vi "MeasureDarkCurrent.vi"(8 "Multimeter GPIB Address":string, 9 "Amplifier":refnum<visa-resource-name>) -> (0 "Amplifier Error":errorcluster, 1 "Amplifier Settings":T1)   [LabVIEW 2017]
uses:
  Linear Dichroism Controller/AmplifierSettings.ctl
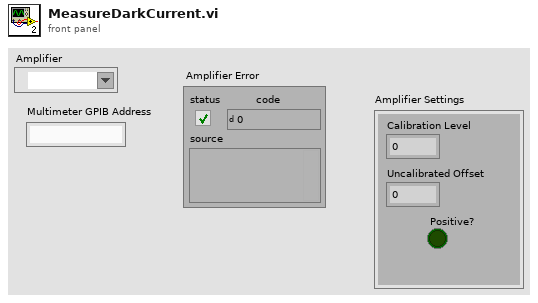
[diagram p1: front panel]
types:
  T1 = typedef "AmplifierSettings.ctl" = cluster{"Calibration Level":dbl, "Uncalibrated Offset":dbl, "Positive?":bool}
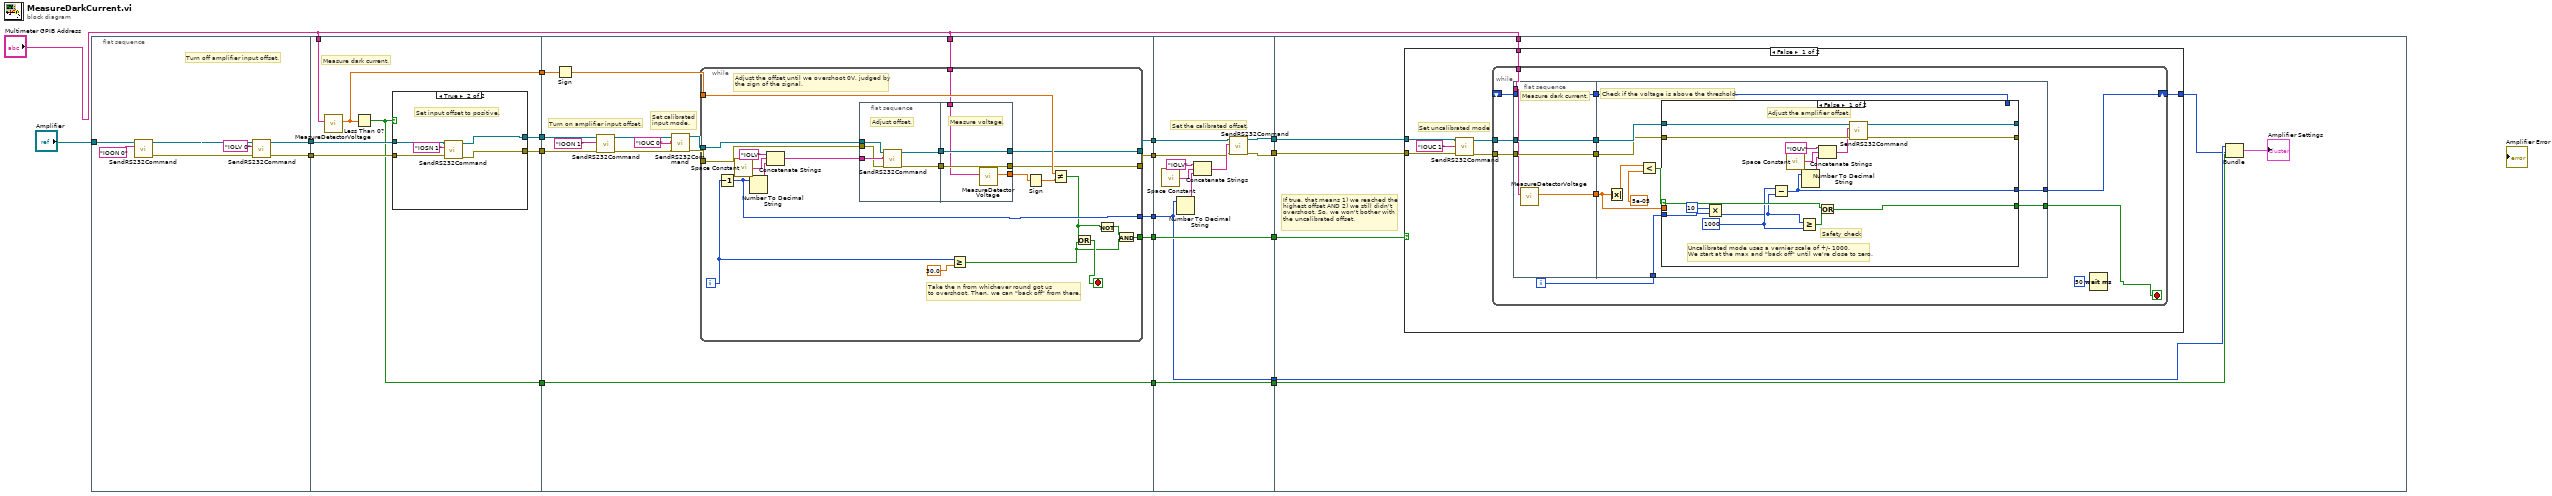
[diagram p0: block diagram]
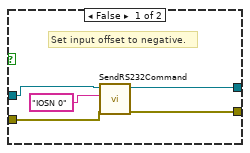
[diagram p2: hidden frame]
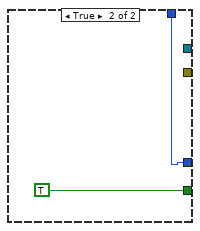
[diagram p3: hidden frame]
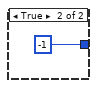
[diagram p4: hidden frame]
diagram:
  n1 = flat-sequence {
    tunnel: "Amplifier" -> [w25]
    tunnel: [w23] -> w17
    tunnel: [w22] -> w16
    tunnel: w17 -> [w32]
    tunnel: w16 -> [w31]
    tunnel: [w30] -> w15
    tunnel: [w29] -> w14
    tunnel: [w28] -> w13
    tunnel: "Multimeter GPIB Address" -> [w27]
    tunnel: [w26] -> w1
    tunnel: w15 -> [w57]
    tunnel: w14 -> [w56]
    tunnel: w13 -> [w55]
    tunnel: [w53] -> w12
    tunnel: [w52] -> w11
    tunnel: [w51] -> w10
    tunnel: [w45] -> w6
    tunnel: "Multimeter GPIB Address" -> [w44]
    tunnel: [w43] -> w2
    tunnel: w1 -> [w43]
    tunnel: w12 -> [w95]
    tunnel: w11 -> [w96]
    tunnel: w10 -> [w91]
    tunnel: [w94] -> w9
    tunnel: [w93] -> w8
    tunnel: [w92] -> w7
    tunnel: w6 -> [w92]
    tunnel: [w91] -> w4
    tunnel: [w90] -> w3
    tunnel: w2 -> [w90]
    tunnel: w9 -> [w107]
    tunnel: w8 -> [w108]
    tunnel: w7 -> [w106]
    tunnel: "Multimeter GPIB Address" -> [w105]
    tunnel: w4 -> [w104]
    tunnel: w3 -> [w102]
    frame #0 {
      # "Turn off amplifier input offset."
      n2 = call "SendRS232Command.vi"("Command"="IOON 0", "VISA/RS232 Device In"=w25) -> ("error out"=w20:errorcluster, "VISA/RS232 Device Out"=w21:refnum<visa-resource-name>)  [unwired: 8 in]
      n3 = call "SendRS232Command.vi"("error in (no error)"=w20, "Command"="IOLV 0", "VISA/RS232 Device In"=w21) -> ("error out"=w22:errorcluster, "VISA/RS232 Device Out"=w23:refnum<visa-resource-name>)  [unwired: 7 in]
    }
    frame #1 {
      # "Measure dark current."
      n4 = call "MeasureDetectorVoltage.vi"("GPIB Address"=w27) -> ("Average Voltage"=w28:dbl)  [unwired: 10 in]
      n5 = Less Than 0?(x=w28) -> (x < 0?=w26:bool)
      n6 = case shown="True" w26 {
        tunnel: w32 -> [w36 w42]
        tunnel: w31 -> [w35 w41]
        tunnel: [w34 w39] -> w30
        tunnel: [w33 w38] -> w29
        frame False {
          # "Set input offset to negative."
          n7 = call "SendRS232Command.vi"("error in (no error)"=w35, "Command"="IOSN 0", "VISA/RS232 Device In"=w36) -> ("error out"=w33:errorcluster, "VISA/RS232 Device Out"=w34:refnum<visa-resource-name>)  [unwired: 7 in]
        }
        frame True {
          # "Set input offset to positive."
          n8 = call "SendRS232Command.vi"("error in (no error)"=w41, "Command"="IOSN 1", "VISA/RS232 Device In"=w42) -> ("error out"=w38:errorcluster, "VISA/RS232 Device Out"=w39:refnum<visa-resource-name>)  [unwired: 7 in]
        }
      }
    }
    frame #2 {
      # "Set calibrated \ninput mode."
      # "Turn on amplifier input offset."
      n9 = Sign(1:w55) -> (0:w54:dbl)
      n10 = call "SendRS232Command.vi"("error in (no error)"=w56, "Command"="IOON 1", "VISA/RS232 Device In"=w57) -> ("error out"=w48:errorcluster, "VISA/RS232 Device Out"=w49:refnum<visa-resource-name>)  [unwired: 7 in]
      n11 = call "SendRS232Command.vi"("error in (no error)"=w48, "Command"="IOUC 0", "VISA/RS232 Device In"=w49) -> ("error out"=w46:errorcluster, "VISA/RS232 Device Out"=w47:refnum<visa-resource-name>)  [unwired: 7 in]
      n12 = while {
        tunnel: w47 -> [w76]
        tunnel: w46 -> [w75]
        tunnel: w54 -> [w71]
        tunnel: [w65] -> w51
        tunnel: [w67] -> w53
        tunnel: [w66] -> w52
        tunnel: [w60] -> w45
        tunnel: w44 -> [w59]
        i -> [w73]
        stop <- w64 stop-if-true
        # "Take the n from whichever round got us \nto overshoot. Then, we can \"back off\" from there."
        # "Adjust the offset until we overshoot 0V, judged by\nthe sign of the signal."
        n13 = Decrement(x=w73) -> (x-1=w65:i32)
        n14 = call <vilib>:"Space Constant.vi"() -> ("String"=w79:string)
        n15 = Number To Decimal String(number=w65) -> (decimal integer string=w78:string)  [unwired: 1 in]
        n16 = Concatenate Strings("IOLV", w79, w78) -> (w77:string)
        n17 = flat-sequence {
          tunnel: w77 -> [w85]
          tunnel: w76 -> [w84]
          tunnel: w75 -> [w83]
          tunnel: [w82] -> w70
          tunnel: [w81] -> w69
          tunnel: [w89] -> w68
          tunnel: w70 -> [w88]
          tunnel: w69 -> [w87]
          tunnel: [w88] -> w67
          tunnel: [w87] -> w66
          tunnel: w59 -> [w86]
          frame #0 {
            # "Adjust offset."
            n18 = call "SendRS232Command.vi"("error in (no error)"=w83, "Command"=w85, "VISA/RS232 Device In"=w84) -> ("error out"=w81:errorcluster, "VISA/RS232 Device Out"=w82:refnum<visa-resource-name>)  [unwired: 7 in]
          }
          frame #1 {
            # "Measure voltage."
            n19 = call "MeasureDetectorVoltage.vi"("GPIB Address"=w86) -> ("Average Voltage"=w89:dbl)  [unwired: 10 in]
          }
        }
        n20 = Greater Or Equal?(x=w73, y=30.0) -> (x >= y?=w61:bool)
        n21 = Sign(1:w68) -> (0:w72:dbl)
        n22 = Not Equal?(x=w71, y=w72) -> (x != y?=w63:bool)
        n23 = Or(x=w63, y=w61) -> (x .or. y?=w64:bool)
        n24 = Not(x=w63) -> (.not. x?=w62:bool)
        n25 = And(x=w62, y=w61) -> (x .and. y?=w60:bool)
      }
    }
    frame #3 {
      # "Set the calibrated offset."
      n26 = call <vilib>:"Space Constant.vi"() -> ("String"=w99:string)
      n27 = Number To Decimal String(number=w91) -> (decimal integer string=w100:string)  [unwired: 1 in]
      n28 = Concatenate Strings("IOLV", w99, w100) -> (w97:string)
      n29 = call "SendRS232Command.vi"("error in (no error)"=w96, "Command"=w97, "VISA/RS232 Device In"=w95) -> ("error out"=w94:errorcluster, "VISA/RS232 Device Out"=w93:refnum<visa-resource-name>)  [unwired: 7 in]
    }
    frame #4 {
      # "If true, that means 1) we reached the \nhighest offset AND 2) we still didn't \novershoot. So, we won't bother with \nthe uncalibrated offset."
      n30 = case shown="False" w106 {
        tunnel: w108 -> [w112 _]
        tunnel: w107 -> [w111 _]
        tunnel: w105 -> [w110 _]
        tunnel: [w109 -1] -> w103
        frame False {
          # "Set uncalibrated mode"
          n31 = call "SendRS232Command.vi"("error in (no error)"=w111, "Command"="IOUC 1", "VISA/RS232 Device In"=w112) -> ("error out"=w114:errorcluster, "VISA/RS232 Device Out"=w115:refnum<visa-resource-name>)  [unwired: 7 in]
          n32 = while {
            tunnel: w115 -> [w125]
            tunnel: w114 -> [w123]
            tunnel: w110 -> [w119]
            shift-right: [w118] -> w109
            shift-left: _ -> [w116]
            i -> [w122]
            stop <- w121 stop-if-true
            n33 = flat-sequence {
              tunnel: [w132] -> w127
              tunnel: [w131] -> w126
              tunnel: w125 -> [w131]
              tunnel: [w130] -> w124
              tunnel: w123 -> [w130]
              tunnel: w119 -> [w129]
              tunnel: [w128] -> w117
              tunnel: w116 -> [w128]
              tunnel: w127 -> [w139]
              tunnel: [w138] -> w121
              tunnel: w126 -> [w137]
              tunnel: w124 -> [w136]
              tunnel: w122 -> [w135]
              tunnel: [w134] -> w118
              tunnel: w117 -> [w133]
              frame #0 {
                # "Measure dark current."
                n34 = call "MeasureDetectorVoltage.vi"("GPIB Address"=w129) -> ("Average Voltage"=w132:dbl)  [unwired: 10 in]
              }
              frame #1 {
                # "Check if the voltage is above the threshold."
                n35 = Absolute Value(x=w139) -> (abs(x)=w142:dbl)
                n36 = Less?(x=w142, y=5e-05) -> (x < y?=w140:bool)
                n37 = case shown="False" w140 {
                  selector: w140 -> [w149 _]
                  tunnel: w139 -> [_ _]
                  tunnel: [w150 TRUE] -> w138
                  tunnel: w137 -> [w158 _]
                  tunnel: w136 -> [w157 _]
                  tunnel: w135 -> [w147 _]
                  tunnel: [w152 _] -> _
                  tunnel: [w151 _] -> _
                  tunnel: [w143 w159] -> w134
                  tunnel: w133 -> [_ w159]
                  frame False {
                    w146 = 1000
                    # "Safety check"
                    # "Uncalibrated mode uses a vernier scale of +/- 1000. \nWe start at the max and \"back off\" until we're close to zero."
                    # "Adjust the amplifier offset."
                    n38 = Multiply(x=10, y=w147) -> (x*y=w145:i32)
                    n39 = Subtract(x=w146, y=w145) -> (x-y=w143:i32)
                    n40 = call <vilib>:"Space Constant.vi"() -> ("String"=w155:string)
                    n41 = Greater Or Equal?(x=w145, y=w146) -> (x >= y?=w148:bool)
                    n42 = Number To Decimal String(number=w143) -> (decimal integer string=w154:string)  [unwired: 1 in]
                    n43 = Concatenate Strings("IOUV", w155, w154) -> (w153:string)
                    n44 = Or(x=w149, y=w148) -> (x .or. y?=w150:bool)
                    n45 = call "SendRS232Command.vi"("error in (no error)"=w157, "Command"=w153, "VISA/RS232 Device In"=w158) -> ("error out"=w151:errorcluster, "VISA/RS232 Device Out"=w152:refnum<visa-resource-name>)  [unwired: 7 in]
                  }
                  frame True {
                  }
                }
              }
            }
            n46 = Wait (ms)(milliseconds to wait=u32 50) -> ()  [unwired: 1 out]
          }
        }
        frame True {
        }
      }
      n47 = Bundle(w104, w103, w102) -> (→"Amplifier Settings":cluster{i32, i32, bool})  [unwired: 1 in]
    }
  }
